vi "Untitled 1 (rosWrite).vi"(8 "error in (no error)":errorcluster, 10 "msg in":string, 11 "ROS in":T1) -> (3 "ROS out":T1={"topic port"=0, "Node"="", "topic"="", "type"="", "node port"=0, "error "={"status"=FALSE, "code"=0, "source"=""}, "Direction"=enum."Node", "Update (ms)"=1, "FIFO size"=1})   [LabVIEW 2016]
uses:
  builds/UnicornMain/UnicornRIO1/ROS for LabVIEW/home/lvuser/natinst/bin/user.lib/ROS for LabVIEW Software/ROS/Code/SubVIs/_ROSControl.ctl
  builds/UnicornMain/UnicornRIO1/ROS for LabVIEW/home/lvuser/natinst/bin/user.lib/ROS for LabVIEW Software/ROS/Code/SubVIs/_ROSDirection.ctl
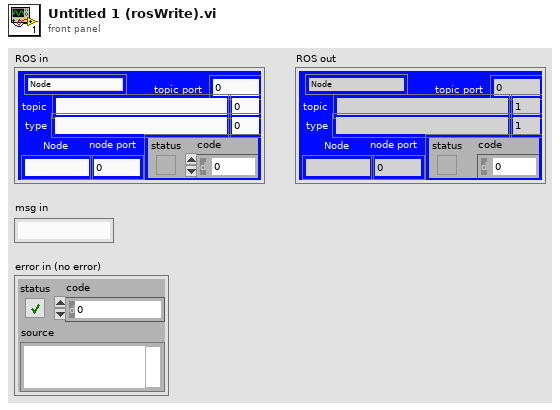
[diagram p1: front panel]
types:
  T1 = typedef "_ROSControl.ctl" = cluster{"topic port":u16, "Node":string, "topic":string, "type":string, "node port":u16, "error ":errorcluster, "Direction":T2, "Update (ms)":u16, "FIFO size":u16}
  T2 = typedef "_ROSDirection.ctl" = enum16{"Node", "Publisher", "Subscriber", "ServiceClient", "ServiceProvider"}
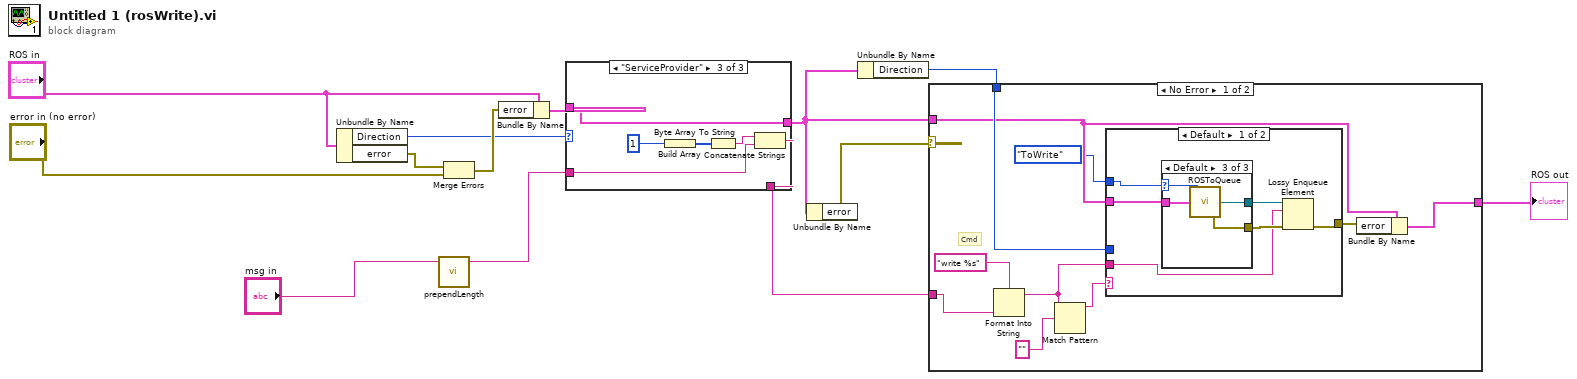
[diagram p0: block diagram]
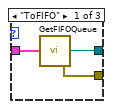
[diagram p2: hidden frame]
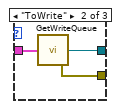
[diagram p3: hidden frame]
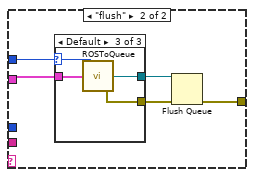
[diagram p4: hidden frame]
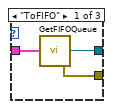
[diagram p5: hidden frame]
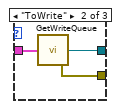
[diagram p6: hidden frame]
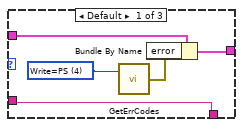
[diagram p8: hidden frame]
diagram:
  n1 = Unbundle By Name("ROS in") -> ("Direction"=w7:T2, "error"=w8:errorcluster)
  n2 = call "prependLength.vi"("msg in"="msg in") -> ("msg out"=w13:string)  [unwired: 4 in]
  n3 = Merge Errors(w8, "error in (no error)") -> (w9:errorcluster)
  n4 = Bundle By Name(cluster="ROS in", "error"=w9) -> (w11:T1)
  n5 = case shown="\"ServiceProvider\"" w7 {
    tunnel: [w17 w20 w22] -> w3
    tunnel: w11 -> [w16 w20 w22]
    tunnel: w13 -> [w14 w19 w24]
    tunnel: [w14 w19 w23] -> w2
    frame Default {
      w18 = u16 4 items=["TopicReadTimeout", "Read=SS", "GetQueueErr", "NoMaster", "Write=PS"] ("Error")
      n6 = call "GetErrCodes.vi"("Error"=w18) -> ("Error"=w15:errorcluster)  [unwired: 1 in]
      n7 = Bundle By Name(cluster=w16, "error"=w15) -> (w17:T1)
    }
    frame "Publisher", "ServiceClient" {
    }
    frame "ServiceProvider" {
      n8 = Build Array(u8 1 ("Numeric")) -> (w26:u8[])
      n9 = Byte Array To String(unsigned byte array=w26) -> (string=w25:string)
      n10 = Concatenate Strings(w25, w24) -> (w23:string)
    }
  }
  n11 = Unbundle By Name(w3) -> ("error"=w5:errorcluster)
  n12 = Unbundle By Name(w3) -> ("Direction"=w4:T2)
  n13 = case shown="No Error" w5 {
    tunnel: w4 -> [w36 _]
    tunnel: w3 -> [w31 w68]
    tunnel: [w32 w68] -> w1
    tunnel: w2 -> [w28 _]
    frame No Error {
      # "Cmd"
      n14 = Format Into String(format string="write %s", w28) -> (resulting string=w27:string)  [unwired: 2 in, 1 out]
      n15 = Match Pattern(string=w27, regular expression="") -> (before substring=w34:string)  [unwired: 1 in, 3 out]
      n16 = case shown="Default" w34 {
        tunnel: w36 -> [_ _]
        tunnel: w27 -> [w39 _]
        tunnel: enum16{"topic", "node", "ToFIFO", "ToWrite"}."ToWrite" ("Type") -> [w42 w57]
        tunnel: w31 -> [w38 w53]
        tunnel: [w37 w54] -> w33
        frame Default {
          n17 = case shown="Default" w42 {
            selector: w42 -> [_ _ w50]
            tunnel: w38 -> [w45 w48 w52]
            tunnel: [w44 w46 w51] -> w41
            tunnel: [w43 w47 w49] -> w40
            frame "ToFIFO" {
              n18 = call "GetFIFOQueue.vi"("ROS"=w45) -> ("error out"=w43:errorcluster, "queue out"=w44:refnum<queue>)  [unwired: 3 in]
            }
            frame "ToWrite" {
              n19 = call "GetWriteQueue.vi"("ROS"=w48) -> ("error out"=w47:errorcluster, "queue out"=w46:refnum<queue>)  [unwired: 3 in]
            }
            frame Default {
              n20 = call "ROSToQueue.vi"("ROS"=w52, "Name"=w50) -> ("error out"=w49:errorcluster, "queue"=w51:refnum<queue>)  [unwired: 2 in]
            }
          }
          n21 = Lossy Enqueue Element(queue=w41, element=w39, error in (no error)=w40) -> (error out=w37:errorcluster)  [unwired: 3 out]
        }
        frame "flush" {
          n22 = case shown="Default" w57 {
            selector: w57 -> [_ _ w65]
            tunnel: w53 -> [w60 w63 w67]
            tunnel: [w59 w61 w66] -> w55
            tunnel: [w58 w62 w64] -> w56
            frame "ToFIFO" {
              n23 = call "GetFIFOQueue.vi"("ROS"=w60) -> ("error out"=w58:errorcluster, "queue out"=w59:refnum<queue>)  [unwired: 3 in]
            }
            frame "ToWrite" {
              n24 = call "GetWriteQueue.vi"("ROS"=w63) -> ("error out"=w62:errorcluster, "queue out"=w61:refnum<queue>)  [unwired: 3 in]
            }
            frame Default {
              n25 = call "ROSToQueue.vi"("ROS"=w67, "Name"=w65) -> ("error out"=w64:errorcluster, "queue"=w66:refnum<queue>)  [unwired: 2 in]
            }
          }
          n26 = Flush Queue(queue=w55, error in (no error)=w56) -> (error out=w54:errorcluster)  [unwired: 2 out]
        }
      }
      n27 = Bundle By Name(cluster=w31, "error"=w33) -> (w32:T1)
    }
    frame Error {
    }
  }
  "ROS out" <- w1
